vi "Get_fast_channels.vi"(1 "uint16s":u64[](array[numeric])) -> (0 "Fast channels":T1(array[cluster]))   [LabVIEW 2013]
panel:
  out "Array":i32[](array[numeric])
  out "size(s)":i32
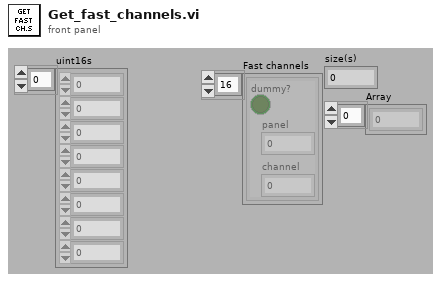
[diagram p1: front panel]
types:
  T1 = cluster{"dummy?":bool, "panel":u8, "channel":u8}[]
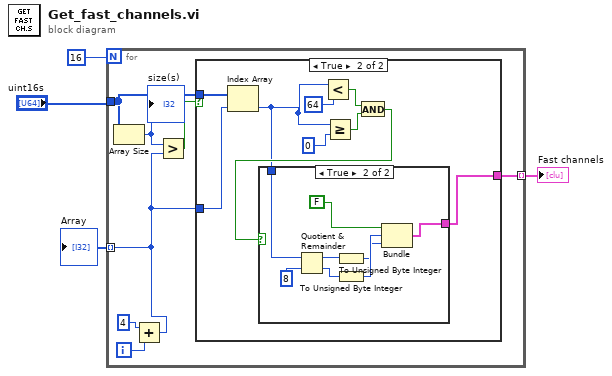
[diagram p0: block diagram]
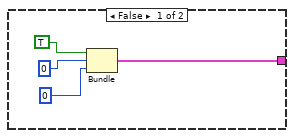
[diagram p2: hidden frame]
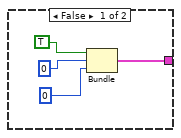
[diagram p3: hidden frame]
diagram:
  n1 = for {
    N: 16 -> [_]
    tunnel: "uint16s" -> [w9]
    tunnel: [w6] -> w2 mode=indexing
    tunnel: [w5] -> w1 mode=indexing
    i -> [w10]
    n2 = Array Size(array=w9) -> (size(s)=w8:i32)
    "size(s)" <- w8
    n3 = Add(x=4, y=w10) -> (x+y=w5:i32)
    n4 = Greater?(x=w8, y=w5) -> (0:w7:bool)
    n5 = case shown="True" w7 {
      tunnel: w9 -> [_ w20]
      tunnel: [w12 w18] -> w6
      tunnel: w5 -> [_ w16]
      frame False {
        n6 = Bundle("dummy?"=TRUE, "panel"=u8 0, "channel"=u8 0) -> (w12:cluster{"dummy?":bool, "panel":u8, "channel":u8})  [unwired: 1 in]
      }
      frame True {
        n7 = Index Array(array=w20, index=w16) -> (element=w17:u64)
        n8 = Less?(x=w17, y=64) -> (x < y?=w21:bool)
        n9 = Greater Or Equal?(x=w17, y=0) -> (x >= y?=w22:bool)
        n10 = And(x=w21, y=w22) -> (x .and. y?=w19:bool)
        n11 = case shown="True" w19 {
          tunnel: [w25 w29] -> w18
          tunnel: w17 -> [_ w30]
          frame False {
            n12 = Bundle("dummy?"=TRUE, "panel"=u8 0, "channel"=u8 0) -> (w25:cluster{"dummy?":bool, "panel":u8, "channel":u8})  [unwired: 1 in]
          }
          frame True {
            n13 = Quotient & Remainder(x=w30, y=8) -> (x-y*floor(x/y)=w35:u64, floor(x/y)=w34:u64)
            n14 = To Unsigned Byte Integer(number=w35) -> (unsigned 8bit integer=w31:u8)
            n15 = To Unsigned Byte Integer(number=w34) -> (unsigned 8bit integer=w32:u8)
            n16 = Bundle("dummy?"=FALSE, w32, w31) -> (w29:cluster{"dummy?":bool, u8, u8})  [unwired: 1 in]
          }
        }
      }
    }
  }
  "Fast channels" <- w2
  "Array" <- w1
